vi "MKS MF1 USB.vi"() -> ()   [LabVIEW 2015]
doc: "Example VI that demonstrates all library features."
uses:
  PL MKS MF1 USB.lvclass
panel:
  in  "autozero":bool
  in  "wink":bool
  in  "gas table index":u8
  out "temperature, °C":dbl
  out "valve, %":dbl
  out "measured flow rate":dbl
  in  "flow rate setpoint":dbl
  in  "valve mode":u8(ring) items=["normal", "closed", "purge"]
  out "error status":T1
  out "status":T2
  in  "address":u8=1
  in  "parity":enum16{"None", "Odd", "Even", "Mark", "Space"}(ring)
  out "MKS MF1":refnum<class "PL MKS MF1 USB.lvclass">
  in  "port":refnum<visa-resource-name>
  in  "stop bits":u16(ring)=10 items=["1.0"=10, "1.5"=15, "2.0"=20]
  in  "data bits":u16=8
  in  "baud rate":u32=115200
  out "error":errorcluster
  in  "stop":bool
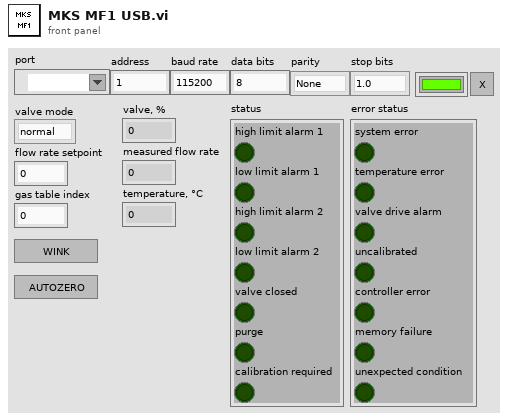
[diagram p1: front panel]
types:
  T1 = cluster{"system error":bool, "temperature error":bool, "valve drive alarm":bool, "uncalibrated":bool, "controller error":bool, "memory failure":bool, "unexpected condition":bool}
  T2 = cluster{"high limit alarm 1":bool, "low limit alarm 1":bool, "high limit alarm 2":bool, "low limit alarm 2":bool, "valve closed":bool, "purge":bool, "calibration required":bool}
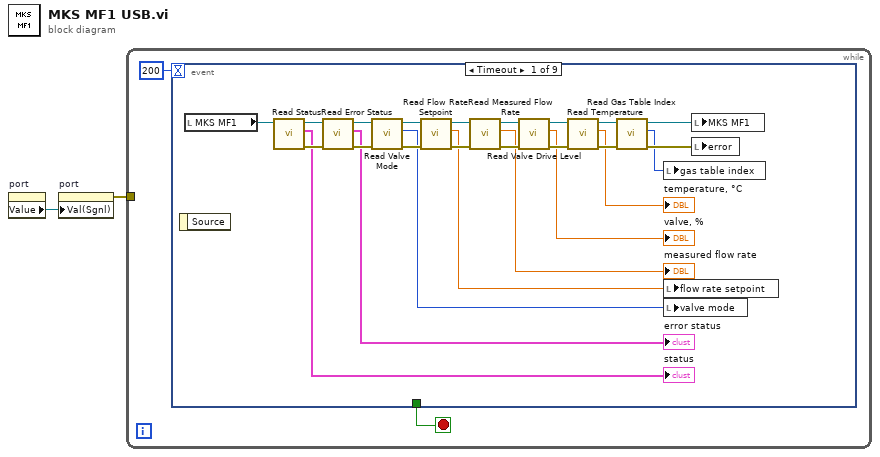
[diagram p0: block diagram]
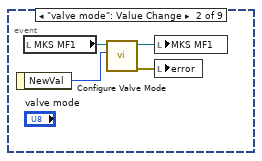
[diagram p2: hidden frame]
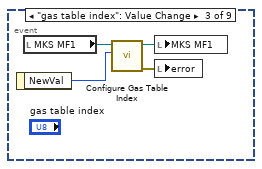
[diagram p3: hidden frame]
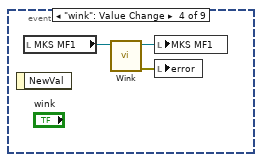
[diagram p4: hidden frame]
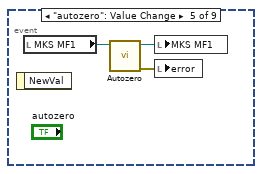
[diagram p5: hidden frame]
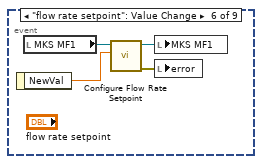
[diagram p6: hidden frame]
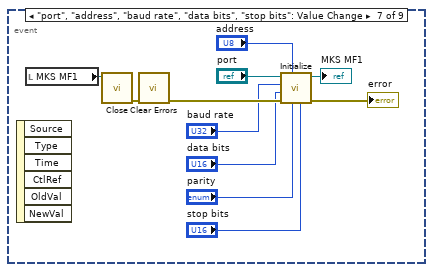
[diagram p7: hidden frame]
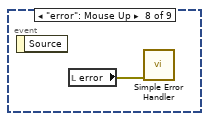
[diagram p8: hidden frame]
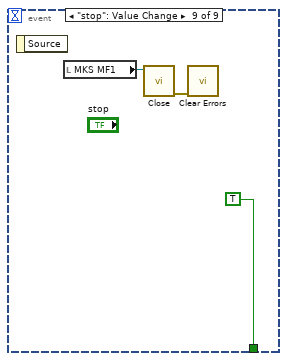
[diagram p9: hidden frame]
diagram:
  n1 = property on="port" class="VISAName"() -> ("Value"=w1:refnum<visa-resource-name>)  [unwired: 2 in, 2 out]
  n2 = property on="port" class="VISAName"("Val(Sgnl)"=w1) -> (error out=w2:errorcluster)  [unwired: 2 in, 1 out]
  n3 = while {
    tunnel: w2 -> [_]
    stop <- w3 stop-if-true
    n4 = event shown="[0] Timeout" {
      selector: _ -> [_ _ _ _ _ _ _ _ _]
      dyn-events: _ -> [_ _ _ _ _ _ _ _ _]
      timeout: 200 -> [_ _ _ _ _ _ _ _ _]
      tunnel: [_ _ _ _ _ _ _ _ TRUE ("stop")] -> w3
      event Timeout {
        n5 = event-data() -> ()  [unwired: 1 in, 1 out]
        n6 = local read "MKS MF1"() -> (w29:refnum<class "PL MKS MF1 USB.lvclass">)
        n7 = call "Read Status.vi"("MKS MF1 in"=w29) -> ("error out"=w19:errorcluster, "status"=→"status":T2, "MKS MF1 out"=w20:refnum<class "PL MKS MF1 USB.lvclass">)  [unwired: 8 in]
        n8 = call "Read Error Status.vi"("error in (no error)"=w19, "MKS MF1 in"=w20) -> ("error out"=w18:errorcluster, "error status"=→"error status":T1, "MKS MF1 out"=w21:refnum<class "PL MKS MF1 USB.lvclass">)  [unwired: 7 in]
        n9 = call "Read Valve Mode.vi"("error in (no error)"=w18, "MKS MF1 in"=w21) -> ("error out"=w17:errorcluster, "valve mode"=w10:u8, "MKS MF1 out"=w22:refnum<class "PL MKS MF1 USB.lvclass">)  [unwired: 7 in]
        n10 = call "Read Flow Rate Setpoint.vi"("error in (no error)"=w17, "MKS MF1 in"=w22) -> ("error out"=w16:errorcluster, "flow rate setpoint, calibrated flow unit"=w5:dbl, "MKS MF1 out"=w23:refnum<class "PL MKS MF1 USB.lvclass">)  [unwired: 7 in]
        n11 = call "Read Measured Flow Rate.vi"("error in (no error)"=w16, "MKS MF1 in"=w23) -> ("error out"=w15:errorcluster, "measured flow rate, calibrated flow unit"=→"measured flow rate":dbl, "MKS MF1 out"=w24:refnum<class "PL MKS MF1 USB.lvclass">)  [unwired: 7 in]
        n12 = call "Read Valve Drive Level.vi"("error in (no error)"=w15, "MKS MF1 in"=w24) -> ("error out"=w14:errorcluster, "valve drive level, %"=→"valve, %":dbl, "MKS MF1 out"=w25:refnum<class "PL MKS MF1 USB.lvclass">)  [unwired: 7 in]
        n13 = call "Read Temperature.vi"("error in (no error)"=w14, "MKS MF1 in"=w25) -> ("error out"=w13:errorcluster, "temperature, °C"=→"temperature, °C":dbl, "MKS MF1 out"=w26:refnum<class "PL MKS MF1 USB.lvclass">)  [unwired: 7 in]
        n14 = call "Read Gas Table Index.vi"("error in (no error)"=w13, "MKS MF1 in"=w26) -> ("error out"=w27:errorcluster, "gas table index"=w6:u8, "MKS MF1 out"=w28:refnum<class "PL MKS MF1 USB.lvclass">)  [unwired: 7 in]
        n15 = local write "gas table index"(w6) -> ()
        n16 = local write "flow rate setpoint"(w5) -> ()
        n17 = local write "valve mode"(w10) -> ()
        n18 = local write "MKS MF1"(w28) -> ()
        n19 = local write "error"(w27) -> ()
      }
      event "valve mode": Value Change {
        n20 = event-data() -> ("NewVal"=w32:u8)  [unwired: 1 in]
        n21 = local read "MKS MF1"() -> (w33:refnum<class "PL MKS MF1 USB.lvclass">)
        n22 = call "Configure Valve Mode.vi"("valve mode"=w32, "MKS MF1 in"=w33) -> ("error out"=w30:errorcluster, "MKS MF1 out"=w31:refnum<class "PL MKS MF1 USB.lvclass">)  [unwired: 8 in]
        n23 = local write "MKS MF1"(w31) -> ()
        n24 = local write "error"(w30) -> ()
      }
      event "gas table index": Value Change {
        n25 = event-data() -> ("NewVal"=w34:u8)  [unwired: 1 in]
        n26 = local read "MKS MF1"() -> (w35:refnum<class "PL MKS MF1 USB.lvclass">)
        n27 = call "Configure Gas Table Index.vi"("gas table index"=w34, "MKS MF1 in"=w35) -> ("error out"=w36:errorcluster, "MKS MF1 out"=w37:refnum<class "PL MKS MF1 USB.lvclass">)  [unwired: 8 in]
        n28 = local write "MKS MF1"(w37) -> ()
        n29 = local write "error"(w36) -> ()
      }
      event "wink": Value Change {
        n30 = event-data() -> ()  [unwired: 1 in, 1 out]
        n31 = local read "MKS MF1"() -> (w38:refnum<class "PL MKS MF1 USB.lvclass">)
        n32 = call "Wink.vi"("MKS MF1 in"=w38) -> ("error out"=w39:errorcluster, "MKS MF1 out"=w40:refnum<class "PL MKS MF1 USB.lvclass">)  [unwired: 9 in]
        n33 = local write "MKS MF1"(w40) -> ()
        n34 = local write "error"(w39) -> ()
      }
      event "autozero": Value Change {
        n35 = event-data() -> ()  [unwired: 1 in, 1 out]
        n36 = local read "MKS MF1"() -> (w43:refnum<class "PL MKS MF1 USB.lvclass">)
        n37 = call "Autozero.vi"("MKS MF1 in"=w43) -> ("error out"=w41:errorcluster, "MKS MF1 out"=w42:refnum<class "PL MKS MF1 USB.lvclass">)  [unwired: 9 in]
        n38 = local write "MKS MF1"(w42) -> ()
        n39 = local write "error"(w41) -> ()
      }
      event "flow rate setpoint": Value Change {
        n40 = event-data() -> ("NewVal"=w44:dbl)  [unwired: 1 in]
        n41 = local read "MKS MF1"() -> (w45:refnum<class "PL MKS MF1 USB.lvclass">)
        n42 = call "Configure Flow Rate Setpoint.vi"("flow rate setpoint, calibrated flow unit"=w44, "MKS MF1 in"=w45) -> ("error out"=w46:errorcluster, "MKS MF1 out"=w47:refnum<class "PL MKS MF1 USB.lvclass">)  [unwired: 8 in]
        n43 = local write "MKS MF1"(w47) -> ()
        n44 = local write "error"(w46) -> ()
      }
      event "port", "address", "baud rate", "data bits", "stop bits": Value Change {
        n45 = event-data() -> ()  [unwired: 1 in, 6 out]
        n46 = local read "MKS MF1"() -> (w58:refnum<class "PL MKS MF1 USB.lvclass">)
        n47 = call "Close.vi"("MKS MF1 in"=w58) -> ("error out"=w52:errorcluster)  [unwired: 10 in]
        n48 = call <vilib>:"Clear Errors.vi"("error in (no error)"=w52) -> ("error out"=w56:errorcluster)  [unwired: 5 in, 1 out]
        n49 = call "Initialize.vi"("stop bits (1.0)"="stop bits", "parity (none)"="parity", "address (1)"="address", "error in (no error)"=w56, "data bits (8)"="data bits", "baud rate (115200)"="baud rate", "port"="port") -> ("error out"=→"error":errorcluster, "MKS MF1 out"=→"MKS MF1":refnum<class "PL MKS MF1 USB.lvclass">)  [unwired: 3 in]
      }
      event "error": Mouse Up {
        n50 = event-data() -> ()  [unwired: 1 in, 1 out]
        n51 = local read "error"() -> (w59:errorcluster)
        n52 = call <vilib>:"Simple Error Handler.vi"("error in (no error)"=w59) -> ()  [unwired: 4 in, 5 out]
      }
      event "stop": Value Change {
        n53 = event-data() -> ()  [unwired: 1 in, 1 out]
        n54 = local read "MKS MF1"() -> (w61:refnum<class "PL MKS MF1 USB.lvclass">)
        n55 = call "Close.vi"("MKS MF1 in"=w61) -> ("error out"=w60:errorcluster)  [unwired: 10 in]
        n56 = call <vilib>:"Clear Errors.vi"("error in (no error)"=w60) -> ()  [unwired: 5 in, 2 out]
      }
    }
  }
